vi "Write Active Channel.vi"(8 "error in":errorcluster, 10 "Active Channel":u32, 11 "PRM in":refnum<class "PRM.lvclass">) -> (0 "error out":errorcluster, 3 "PRM out":refnum<class "PRM.lvclass">)   [LabVIEW 2019, in "PRM.lvlib" / "PRM.lvclass"]
uses:
  Library/PRM.lvclass
  Library/PRM.lvclass/PRM.ctl
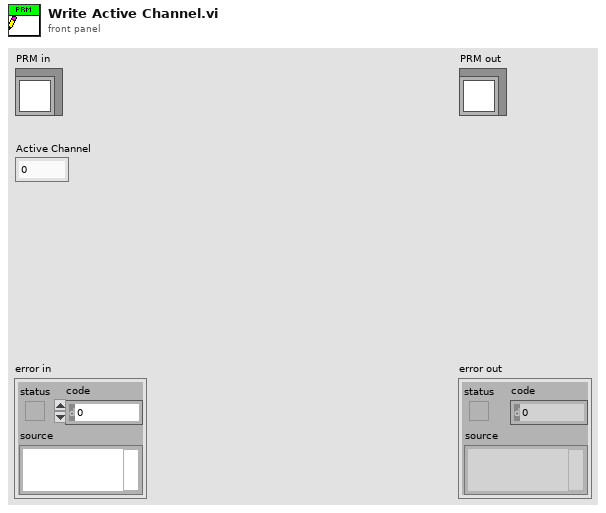
[diagram p1: front panel]
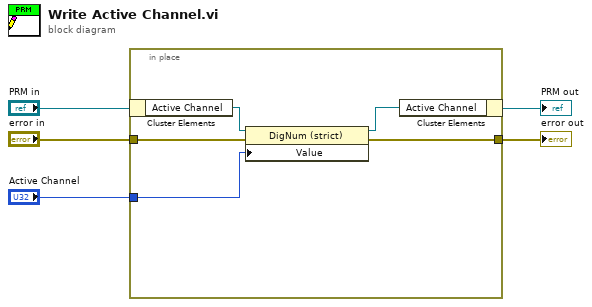
[diagram p0: block diagram]
diagram:
  n1 = in-place {
    in-place-border: "error in" -> [w10]
    in-place-border: [w9] -> w2
    in-place-border: "Active Channel" -> [w6]
    n2 = in-place-cluster #1("PRM in") -> ("Active Channel"=w8:refnum<vi>)
    n3 = property class="DigNum (strict)"(reference=w8, error in=w10, "Value"=w6) -> (reference out=w7:refnum<vi>, error out=w9:errorcluster)
    n4 = in-place-cluster #1("Active Channel"=w7) -> (→"PRM out":refnum<class "PRM.lvclass">)
  }
  "error out" <- w2
